vi "Init.vi"(8 "error in (no error)":errorcluster, 9 "Value":string, 10 "Name":string, 11 "Category":string) -> (0 "error out":errorcluster, 3 "SetProfileParameter out":refnum<class "SetProfileParameter.lvclass">)   [LabVIEW 2020, in "obs-websocket.lvlib" / "SetProfileParameter.lvclass"]
uses:
  SetProfileParameter.lvclass
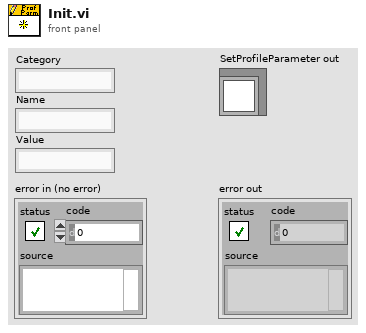
[diagram p1: front panel]
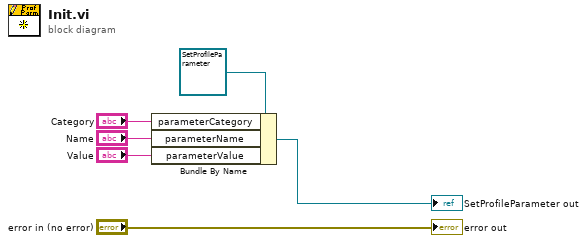
[diagram p0: block diagram]
diagram:
  n1 = Bundle By Name(cluster=refnum<class "SetProfileParameter.lvclass"> refnum ("SetProfileParameter in"), "parameterCategory"="Category", "parameterName"="Name", "parameterValue"="Value") -> (→"SetProfileParameter out":refnum<class "SetProfileParameter.lvclass">)
  "error out" <- "error in (no error)"
